vi "get_hostMessages_p.vi"(0 "MoAgSy_Host":refnum<class "MoAgSy_Host.lvclass">, 5 "error in (no error)":errorcluster) -> (14 "dup MoAgSy_Host":refnum<class "MoAgSy_Host.lvclass">, 16 "Host Messages":refnum<class "MoAgSy_Message.lvclass">[](array[class]), 19 "error out":errorcluster)   [LabVIEW 2009, in "MoAgSy.lvlib" / "MoAgSy_Host.lvclass"]
doc: "<B>protected</B> VI returns internal messages of mobile agent host class.\nIf a message for the host is received, it is enqueued in the internal message array.\nThis VI returns all elements of the array to handle all incoming host messages.\n\nF.Berck@gsi.de\nGSI Darmstadt 2009"
uses:
  MoAgSy_Host.lvclass
  MoAgSy_Message/MoAgSy_Message.lvclass
  MoAgSy_Host.lvclass/MoAgSy_Host.ctl
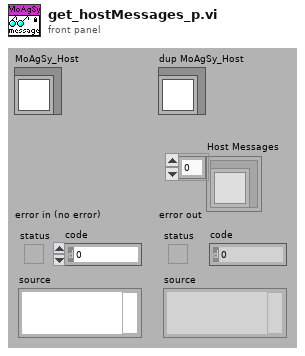
[diagram p1: front panel]
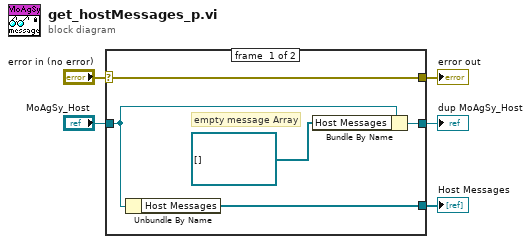
[diagram p0: block diagram]
diagram:
  n1 = case shown="No Error" "error in (no error)" {
    selector: "error in (no error)" -> [w10 w11]
    tunnel: [w10 w11] -> w4
    tunnel: [w7 w12] -> w2
    tunnel: "MoAgSy_Host" -> [w8 w12]
    tunnel: [w9 _] -> w1
    frame #0 {
      # "empty message Array"
      n2 = Unbundle By Name(w8) -> ("Host Messages"=w9:refnum<class "MoAgSy_Message.lvclass">[])
      n3 = Bundle By Name(cluster=w8, "Host Messages"=refnum<class "MoAgSy_Message.lvclass">[] []) -> (w7:refnum<class "MoAgSy_Host.lvclass">)
    }
    frame #1 {
    }
  }
  "error out" <- w4
  "dup MoAgSy_Host" <- w2
  "Host Messages" <- w1
